vi "clearHealthAndStatus.vi"(8 "error in (no error)":errorcluster, 11 "RTHealthAndStatus in":refnum<class "RTHealthAndStatus.lvclass">) -> (0 "error out":errorcluster, 3 "RTHealthAndStatus out":refnum<class "RTHealthAndStatus.lvclass">)   [LabVIEW 2016, in "RTHealthAndStatus.lvlib" / "RTHealthAndStatus.lvclass"]
uses:
  RTHealthAndStatus.lvclass
  RTHealthAndStatus.lvclass/RTHealthAndStatus.ctl
  Common_RT_FPGA/IWriteU64FIFO/IWriteU64FIFO.lvclass
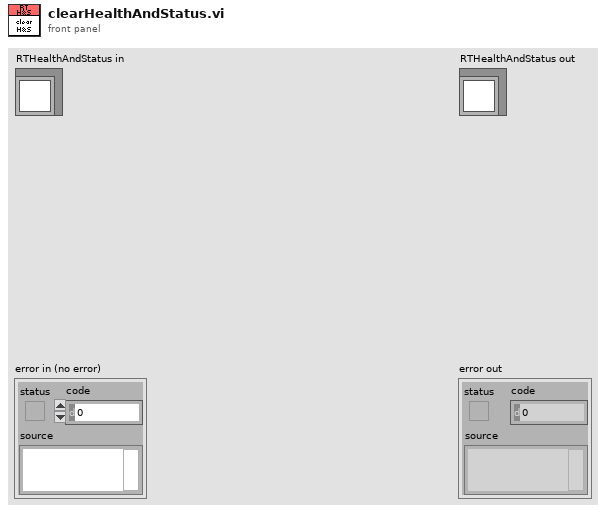
[diagram p1: front panel]
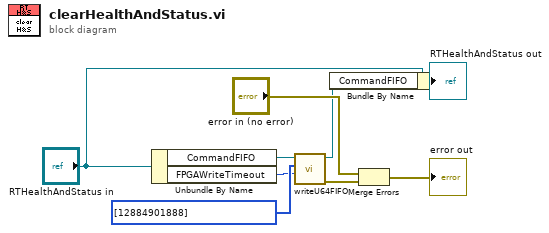
[diagram p0: block diagram]
diagram:
  n1 = Unbundle By Name("RTHealthAndStatus in") -> ("CommandFIFO"=w7:refnum<class "IWriteU64FIFO.lvclass">, "FPGAWriteTimeout"=w5:i32)
  n2 = call-dynamic "writeU64FIFO.vi"("Timeout"=w5, "Data"=u64[] [12884901888], "IWriteU64FIFO in"=w7) -> ("error out"=w4:errorcluster, "IWriteU64FIFO out"=w1:refnum<class "IWriteU64FIFO.lvclass">)  [unwired: 6 in, 1 out]
  n3 = Bundle By Name(cluster="RTHealthAndStatus in", "CommandFIFO"=w1) -> (→"RTHealthAndStatus out":refnum<class "RTHealthAndStatus.lvclass">)
  n4 = Merge Errors("error in (no error)", w4) -> (→"error out":errorcluster)
